vi "camera_waveform.vi"(8 "Resolution":dbl, 9 "Sweep Interval (µS)":u32, 10 "Actual Sweep Time (µS)":u32, 11 "Phase Shift (µS)":i32) -> (2 "Digital Waveform Graph":digitalwaveform(graph))   [LabVIEW 2013]
uses:
  <vilib>/Waveform/DWDTOps.llb/Digital Pattern Generator (Single Value).vi
  <vilib>/Waveform/DWDTOps.llb/DWDT Append Digital Samples.vi
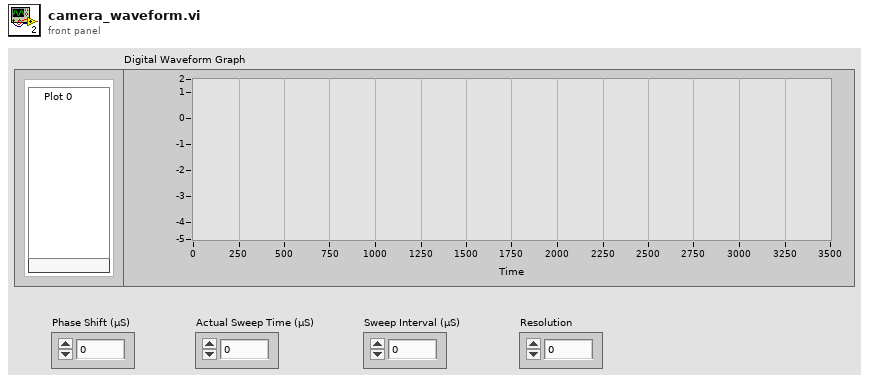
[diagram p1: front panel]
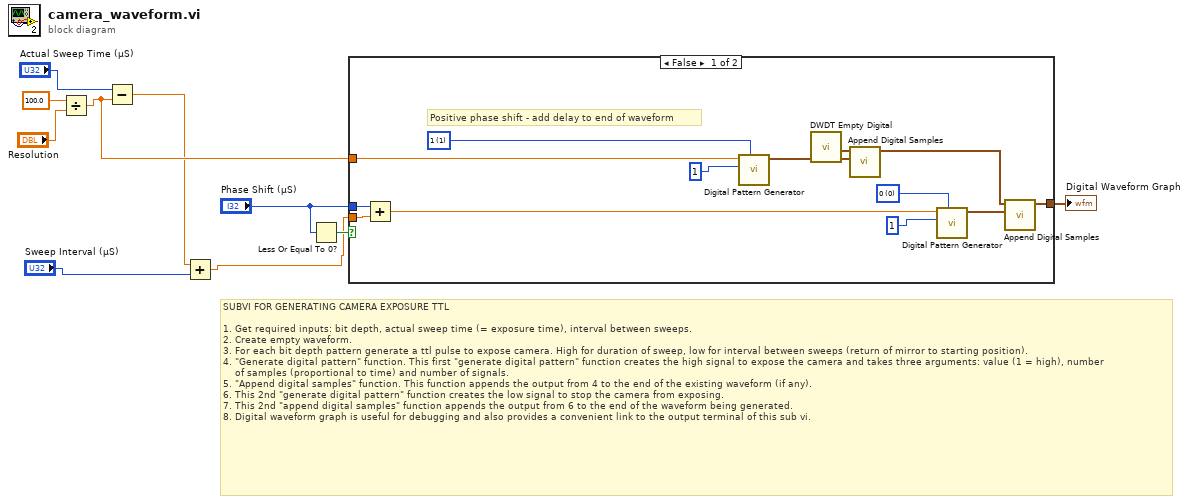
[diagram p0: block diagram]
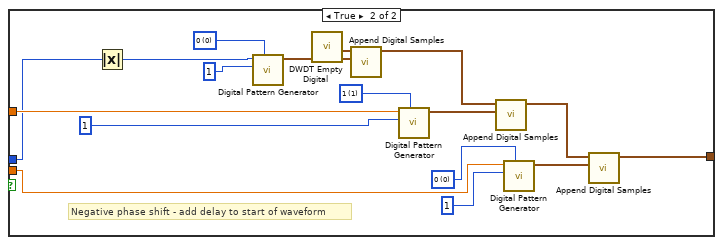
[diagram p2: hidden frame]
diagram:
  # "SUBVI FOR GENERATING CAMERA EXPOSURE TTL\n\n1. Get required inputs: bit depth, actual sweep time (= exposure time), interval between sweeps.\n2. Create empty waveform.\n3. For each bit depth pattern generate a ttl pulse to expose camera. High for duration of sweep, low for interval between sweeps (return of mirror to starting position).\n4. \"Generate digital pattern\" function. This first \"generate digital pattern\" function creates the high signal to expose the camera and takes three arguments: value (1 = high), number \n    of samples (proportional to time) and number of signals.\n5. \"Append digital samples\" function. This function appends the output from 4 to the end of the existing waveform (if any).\n6. This 2nd \"generate digital pattern\" function creates the low signal to stop the camera from exposing.\n7. This 2nd \"append digital samples\" function appends the output from 6 to the end of the waveform being generated.\n8. Digital waveform graph is useful for debugging and also provides a convenient link to the output terminal of this sub vi."
  n1 = Divide(x=100.0, y="Resolution") -> (x/y=w4:dbl)
  n2 = Subtract(x="Actual Sweep Time (µS)", y=w4) -> (x-y=w1:dbl)
  n3 = Add(x=w1, y="Sweep Interval (µS)") -> (x+y=w3:dbl)
  n4 = Less Or Equal To 0?(x="Phase Shift (µS)") -> (x <= 0?=w10:bool)
  n5 = case shown="False" w10 {
    tunnel: "Phase Shift (µS)" -> [w14 w25]
    tunnel: w4 -> [w15 w28]
    tunnel: w3 -> [w13 w27]
    tunnel: [w11 w26] -> w8
    frame False {
      w17 = u8 0 items=["0", "1", "Z", "L", "H", "X", "T", "V"] ("value")
      w20 = u8 1 items=["0", "1", "Z", "L", "H", "X", "T", "V"] ("value")
      # "Positive phase shift - add delay to end of waveform"
      n6 = Add(x=w14, y=w13) -> (x+y=w12:dbl)
      n7 = call-poly <vilib>:"Digital Pattern Generator.vi"("value"=w20, "number of signals"=u32 1, "number of samples"=w15) -> ("digital waveform"=w22:digitalwaveform)  [unwired: 7 in, 1 out]
      n8 = call <vilib>:"DWDT Empty Digital.vi"() -> ("digital waveform out"=w23:digitalwaveform)  [unwired: 5 in]
      n9 = call-poly <vilib>:"Append Digital Samples.vi"("digital waveform B"=w22, "digital waveform A"=w23) -> ("digital waveform out"=w21:digitalwaveform)  [unwired: 8 in, 1 out]
      n10 = call-poly <vilib>:"Digital Pattern Generator.vi"("value"=w17, "number of signals"=u32 1, "number of samples"=w12) -> ("digital waveform"=w18:digitalwaveform)  [unwired: 7 in, 1 out]
      n11 = call-poly <vilib>:"Append Digital Samples.vi"("digital waveform B"=w18, "digital waveform A"=w21) -> ("digital waveform out"=w11:digitalwaveform)  [unwired: 8 in, 1 out]
    }
    frame True {
      w31 = u8 0 items=["0", "1", "Z", "L", "H", "X", "T", "V"] ("value")
      w34 = u8 1 items=["0", "1", "Z", "L", "H", "X", "T", "V"] ("value")
      w37 = u8 0 items=["0", "1", "Z", "L", "H", "X", "T", "V"] ("value")
      # "Negative phase shift - add delay to start of waveform"
      n12 = Absolute Value(x=w25) -> (abs(x)=w24:i32)
      n13 = call-poly <vilib>:"Digital Pattern Generator.vi"("value"=w37, "number of signals"=u32 1, "number of samples"=w24) -> ("digital waveform"=w39:digitalwaveform)  [unwired: 7 in, 1 out]
      n14 = call <vilib>:"DWDT Empty Digital.vi"() -> ("digital waveform out"=w40:digitalwaveform)  [unwired: 5 in]
      n15 = call-poly <vilib>:"Append Digital Samples.vi"("digital waveform B"=w39, "digital waveform A"=w40) -> ("digital waveform out"=w38:digitalwaveform)  [unwired: 8 in, 1 out]
      n16 = call-poly <vilib>:"Digital Pattern Generator.vi"("value"=w34, "number of signals"=u32 1, "number of samples"=w28) -> ("digital waveform"=w35:digitalwaveform)  [unwired: 7 in, 1 out]
      n17 = call-poly <vilib>:"Append Digital Samples.vi"("digital waveform B"=w35, "digital waveform A"=w38) -> ("digital waveform out"=w29:digitalwaveform)  [unwired: 8 in, 1 out]
      n18 = call-poly <vilib>:"Digital Pattern Generator.vi"("value"=w31, "number of signals"=u32 1, "number of samples"=w27) -> ("digital waveform"=w32:digitalwaveform)  [unwired: 7 in, 1 out]
      n19 = call-poly <vilib>:"Append Digital Samples.vi"("digital waveform B"=w32, "digital waveform A"=w29) -> ("digital waveform out"=w26:digitalwaveform)  [unwired: 8 in, 1 out]
    }
  }
  "Digital Waveform Graph" <- w8
